vi "Rec Fetch Integer Data (CR).vi"(6 "error in (no error)":errorcluster, 7 "type":i32, 8 "column index":variant, 9 "command-recordset reference":T1) -> (0 "error out":errorcluster, 1 "data":i32, 3 "command-recordset reference out":T1)   [LabVIEW 2020, in "NI_Database_API.lvlib"]
doc: "Retrieves the data located at the <B>column index</B> of the current record in the recordset identified by the <B>recordset reference</B>. The <B>column index</B> can be either the zero-indexed position of the column in the recordset or the name of the column. Wire data to the <B>type</B> input to determine the polymorphic instance to use or manually select the instance."
uses:
  <vilib>/addons/database/NI_Database_API.lvlib
  <vilib>/addons/database/Command-Recordset.llb/Cmd-Rec Object Reference.ctl
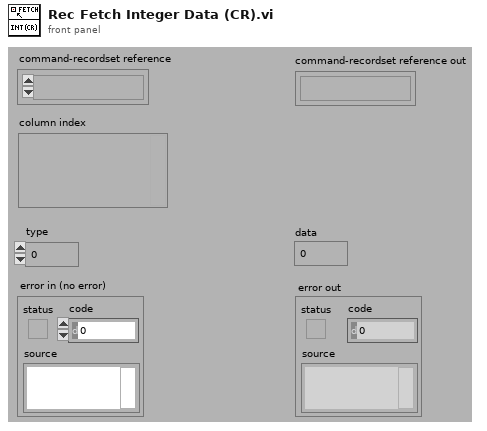
[diagram p1: front panel]
types:
  T1 = typedef "NI_Database_API.lvlib/Cmd-Rec Object Reference.ctl" = refnum<k1>
  T2 = typedef "NI_Database_API.lvlib/Cmd-Rec Data Members.ctl" = cluster{"recordset reference":T3, "command reference":T4}
  T3 = typedef "NI_Database_API.lvlib/Rec ObjectReference.ctl" = refnum<k1>
  T4 = typedef "NI_Database_API.lvlib/Cmd ObjectReference.ctl" = refnum<k1>
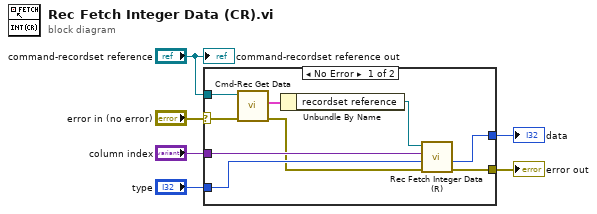
[diagram p0: block diagram]
diagram:
  n1 = case shown="No Error" "error in (no error)" {
    selector: "error in (no error)" -> [w7 w16]
    tunnel: "column index" -> [w14 _]
    tunnel: [w13 w16] -> w5
    tunnel: [w12 _] -> w4
    tunnel: "type" -> [w11 _]
    tunnel: "command-recordset reference" -> [w8 _]
    frame No Error {
      n2 = call <vilib>:"Cmd-Rec Get Data.vi"("error in (no error)"=w7, "command-recordset reference"=w8) -> ("error out"=w9:errorcluster, "data"=w10:T2)  [unwired: 2 in, 2 out]
      n3 = Unbundle By Name(w10) -> ("recordset reference"=w15:T3)
      n4 = call <vilib>:"Rec Fetch Integer Data (R).vi"("error in (no error)"=w9, "type"=w11, "column index"=w14, "recordset reference"=w15) -> ("error out"=w13:errorcluster, "data"=w12:i32)  [unwired: 3 in, 1 out]
    }
    frame Error {
    }
  }
  "data" <- w4
  "error out" <- w5
  "command-recordset reference out" <- "command-recordset reference"
